vi "#6.vi"(0 "System no.":i32=1 min=1 max=4 step=1, 5 "error in":errorcluster) -> (14 "Pos change?":bool[](array[boolean]), 19 "error out":errorcluster)   [LabVIEW 2020]
doc: "Polls for change in position of the connected axes by sending the single ASCII character 6. After a position change #6 answer is reset to FALSE with next POS? query. Connected axes are read from Global2.vi and displayed on the front panel for assignment.\n\nE-517: #6 can be used in open-loop and closed-loop operation.\nThe query considers only motion caused by control sources (e.g. move commands), but ignores position changes caused by amplifier noise.\n\nC-887, F-206: For GCS syntax version = GCS 1.0 (check with CSV?.vi. If CSV?.vi is not supported, syntax version is GCS 1.0), Only first field of Pos change? array is valid, refers to whole system.\n\nC-887, M-8X0: For GCS syntax version = GCS 1.0 (check with CSV?.vi. If CSV?.vi is not supported, syntax version is GCS 1.0), only first field of Pos change? array is valid, refers to whole system."
panel:
  out "Connected axes":string[](array[string])
  # "Polls for change in position of the connected axes."
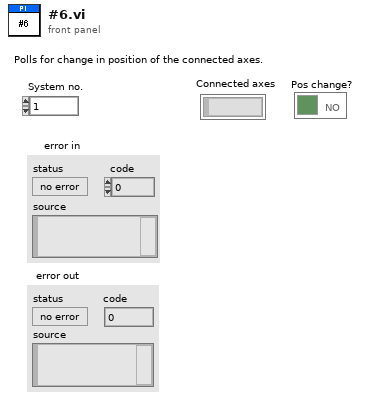
[diagram p1: front panel]
types:
  T1 = enum16{"Disable error check", "Force error check", "Use global settings"}
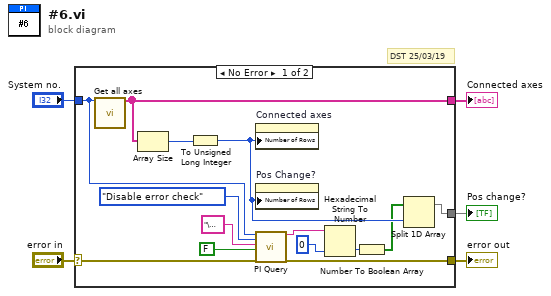
[diagram p0: block diagram]
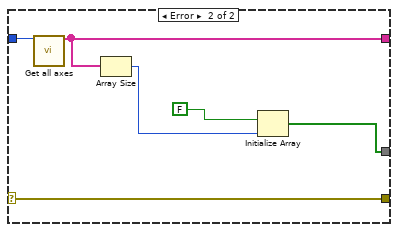
[diagram p2: hidden frame]
diagram:
  # "DST 25/03/19"
  n1 = case shown="No Error" "error in" {
    selector: "error in" -> [w11 w25]
    tunnel: [w8 w20] -> w5
    tunnel: "System no." -> [w15 w24]
    tunnel: [w14 w22] -> w3
    tunnel: [w12 w25] -> w2
    frame No Error {
      n2 = call "Get all axes.vi"("System no."=w15) -> ("Conn. Axes"=w14:string[])  [unwired: 18 out]
      n3 = Array Size(array=w14) -> (size(s)=w17:i32)
      n4 = To Unsigned Long Integer(number=w17) -> (unsigned 32bit integer=w7:u32)
      n5 = property on="Connected axes" class="Arr (strict)"("Number of Rows"=w7) -> ()  [unwired: 2 in, 2 out]
      n6 = property on="Pos Change?" class="Arr (strict)"("Number of Rows"=w7) -> ()  [unwired: 2 in, 2 out]
      n7 = call "PI Query.vi"("System no."=w15, "Error check settings"=T1."Disable error check", "String to send"="\u0006", "Attach termination char.?"=FALSE ("Attach Linefeed?"), "error in"=w11) -> ("String read"=w13:string, "error out"=w12:errorcluster)  [unwired: 2 in, 11 out]
      n8 = Hexadecimal String To Number(string=w13, default (0uL)=u64 0) -> (number=w16:u64)  [unwired: 2 out]
      n9 = Number To Boolean Array(number=w16) -> (Boolean array=w6:bool[])
      n10 = Split 1D Array(array=w6, index=w7) -> (first subarray=w8:bool[])  [unwired: 1 out]
    }
    frame Error {
      n11 = call "Get all axes.vi"("System no."=w24) -> ("Conn. Axes"=w22:string[])  [unwired: 18 out]
      n12 = Array Size(array=w22) -> (size(s)=w21:i32)
      n13 = Initialize Array(FALSE, w21) -> (w20:bool[])
    }
  }
  "error out" <- w2
  "Pos change?" <- w5
  "Connected axes" <- w3
